vi "lxc.vi"() -> ()   [LabVIEW 2017]
uses:
  a005793b-7148-4334-a388-72e6511322f3.vi
panel:
  out "波形图表 4":cluster{dbl, "millisecond timer value":u32}[](graph)
  out "低温  5":bool
  out "高温 5":bool
  in  "停止 10":bool
  out "波形图 2":dbl[](graph)
  out "数组 2":string[](array[string])
  out "波形图表 3":dbl(graph)
  out "波形图表 2":cluster{"y":dbl, "y":dbl, dbl}(graph)
  in  "停止 9":bool
  out "高温 4":bool
  out "低温  4":bool
  out "低温  3":bool
  out "高温 3":bool
  in  "停止 8":bool
  out "波形图表":dbl(graph)
  out "实时温度":cluster{"y":dbl, "y":dbl, dbl}(graph)
  out "下限":bool
  out "上限":bool
  in  "停止 7":bool
  out "x-y":dbl
  in  "停止 6":bool
  in  "停止 5":bool
  out "高温 2":bool
  out "低温  2":bool
  in  "停止 4":bool
  out "已删除元素的数组子集":dbl[](array[numeric])
  out "已删除的部分":dbl[](array[numeric])
  out "重新排序":i32[](array[numeric]) caption="重排后数组"
  out "数组":i32[](array[numeric])
  in  "停止 3":bool
  out "温度 2":dbl
  out "数组 3":dbl[](array[numeric])
  out "温度":dbl
  in  "停止 2":bool
  out "低温":bool
  in  "停止":bool
  out "高温":bool
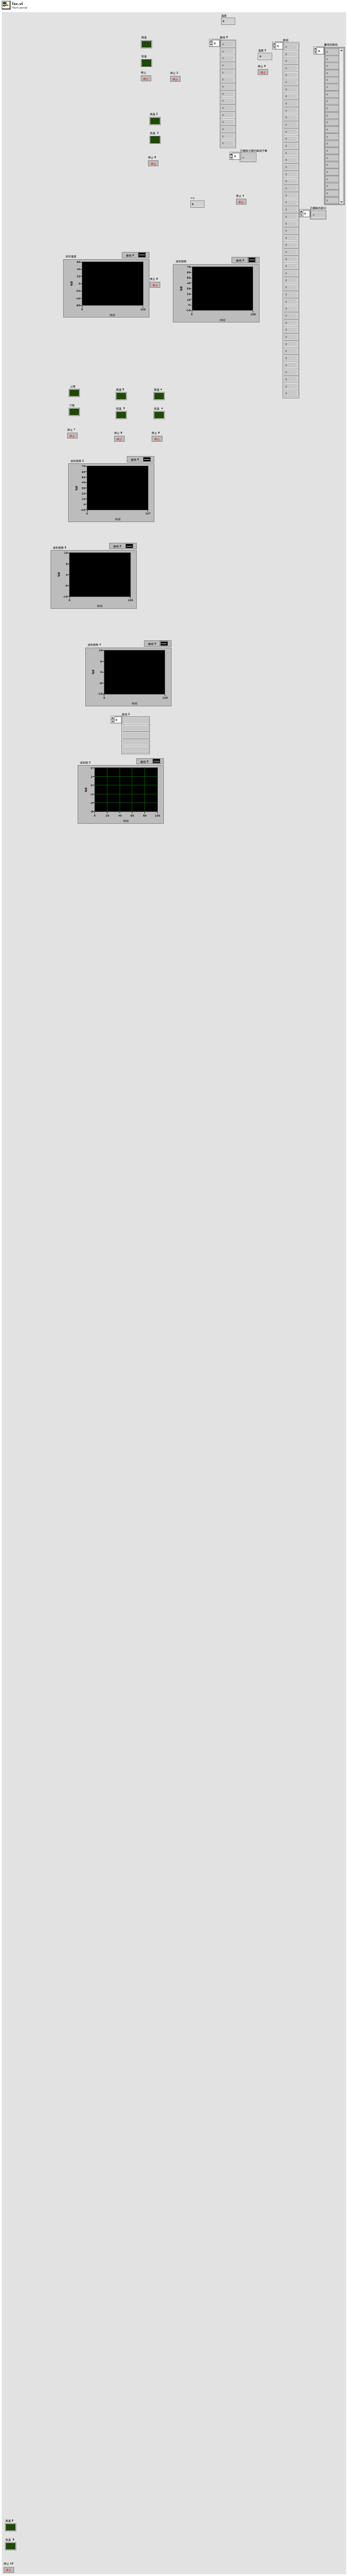
[diagram p1: front panel]
types:
  T1 = enum16{"open", "replace", "create", "open or create", "replace or create", "replace or create with confirmation"}
  T2 = typedef "控件 1.ctl" = i32
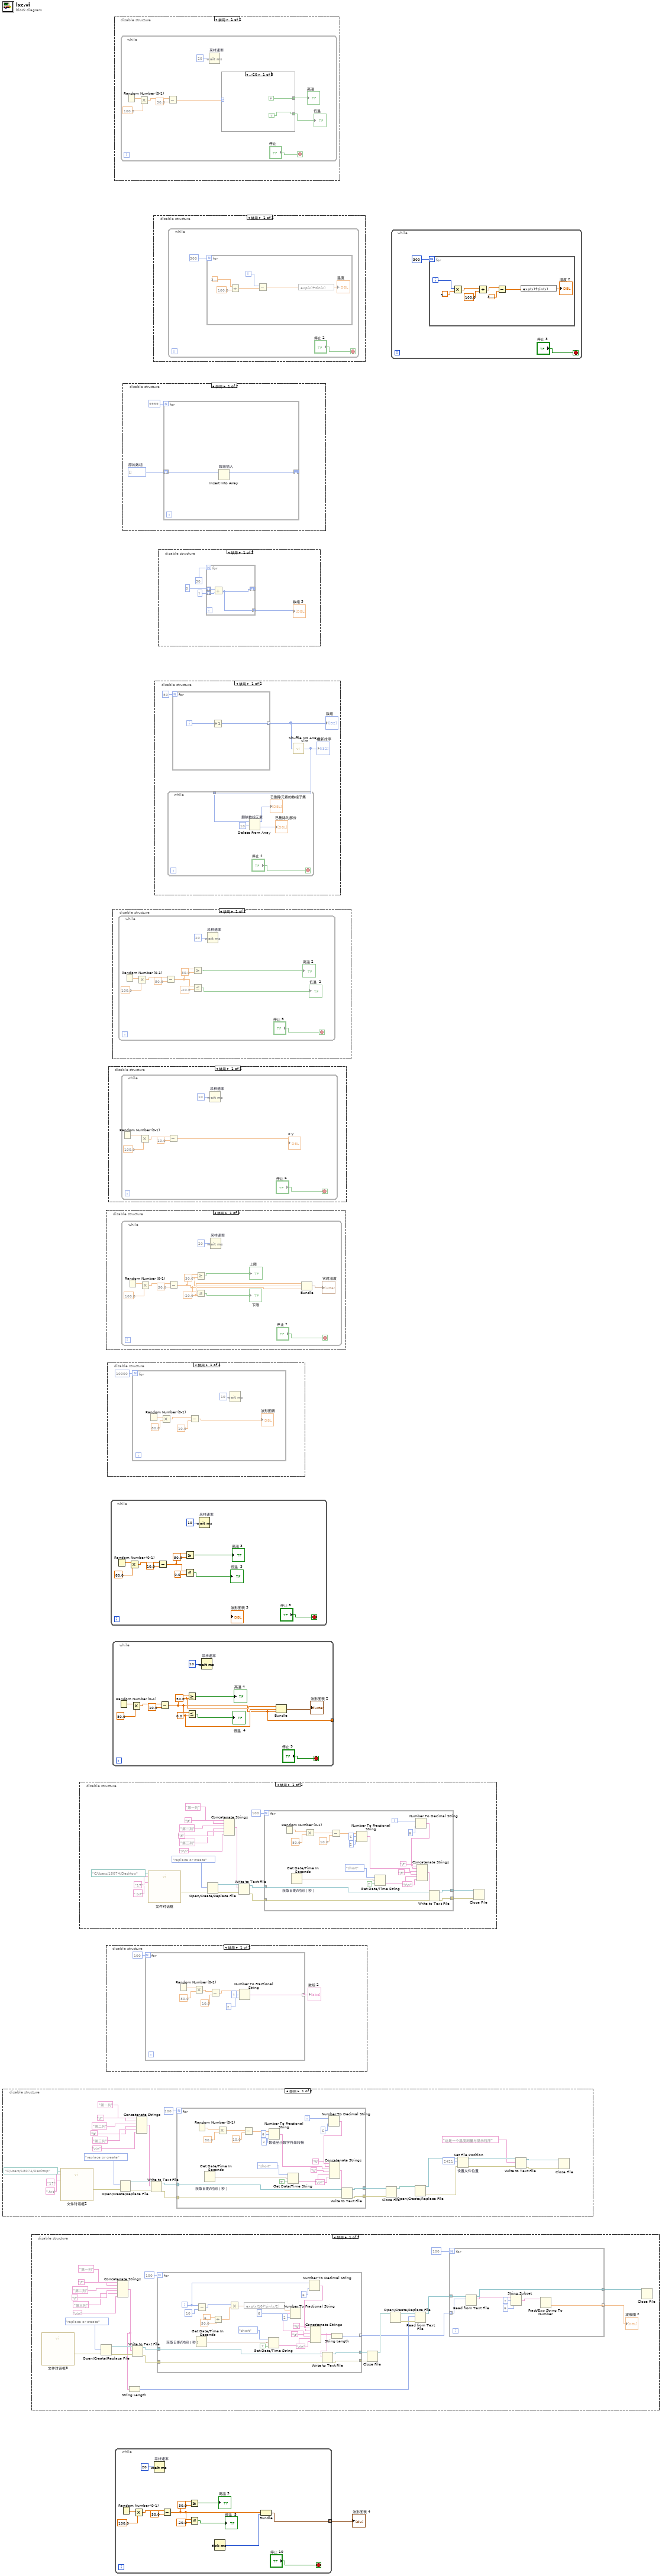
[diagram p0: block diagram]
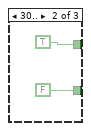
[diagram p14: hidden frame]
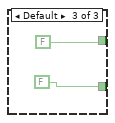
[diagram p15: hidden frame]
diagram:
  n1 = disable-structure shown="禁用" {
    frame Disabled {
      n2 = call "文件对话框2"("start path"=path "C:/Users/18074/Desktop", "default name"="17", "pattern (all files)"=".txt") -> ("error out"=w16:errorcluster)  [unwired: 9 in, 3 out]
      n3 = Open/Create/Replace File(error in=w16, operation (0:open)=T1."replace or create" ("操作(0:open)")) -> (refnum out=w17:refnum<file>, error out=w18:errorcluster)  [unwired: 4 in, 1 out]
      n4 = Concatenate Strings("第一列" ("字符串"), "\t", "第二列" ("字符串"), "\t", "第三列" ("字符串"), "\r\n") -> (w23:string)
      n5 = Write to Text File(file (use dialog)=w17, text=w23, error in=w18) -> (refnum out=w20:refnum<file>, error out=w19:errorcluster)  [unwired: 1 in, 1 out]
      n6 = for {
        N: 100 -> [_]
        tunnel: w20 -> [w48]
        tunnel: w19 -> [w47]
        tunnel: [w37] -> w21
        tunnel: [w36] -> w22
        i -> [w42]
        n7 = Random Number (0-1)() -> (number: 0 to 1=w52:dbl)
        n8 = Get Date/Time In Seconds "获取日期/时间（秒）"() -> (seconds since 1Jan1904=w32:timestamp)
        n9 = Multiply(x=w52, y=80.0) -> (x*y=w50:dbl)
        n10 = Subtract(x=w50, y=10.0) -> (x-y=w45:dbl)
        n11 = Number To Fractional String "数值至小数字符串转换"(number=w45, width (-)=i16 6 ("宽度(-)"), precision (6)=i16 2 ("精度(6)")) -> (F-format string=w39:string)  [unwired: 1 in]
        n12 = Get Date/Time String(date format (0)=enum16{"short", "long", "abbreviated"}."short" ("日期格式(0)"), seconds (now)=w32, want seconds? (F)=TRUE ("UTC格式")) -> (time string=w31:string)  [unwired: 1 out]
        n13 = Number To Decimal String(number=w42, width (-)=i16 6 ("宽度(-)")) -> (decimal integer string=w41:string)
        n14 = Concatenate Strings(w41, "\t", w39, "\t", w31, "\r\n") -> (w35:string)
        n15 = Write to Text File(file (use dialog)=w48, text=w35, error in=w47) -> (refnum out=w37:refnum<file>, error out=w36:errorcluster)  [unwired: 1 in, 1 out]
      }
      n16 = Close File(refnum=w21, error in=w22) -> (path=w10:path)  [unwired: 1 out]
      n17 = Open/Create/Replace File(file path (use dialog)=w10) -> (refnum out=w9:refnum<file>, error out=w8:errorcluster)  [unwired: 5 in, 1 out]
      n18 = Set File Position "设置文件位置"(offset (in bytes) (0)=i64 2421 ("偏移量（字节）（0）"), refnum=w9, error in=w8) -> (refnum out=w7:refnum<file>, error out=w6:errorcluster)  [unwired: 1 in]
      n19 = Write to Text File(file (use dialog)=w7, text="这是一个温度测量与显示程序" ("文本"), error in=w6) -> (refnum out=w4:refnum<file>, error out=w3:errorcluster)  [unwired: 1 in, 1 out]
      n20 = Close File(refnum=w4, error in=w3) -> ()  [unwired: 2 out]
    }
    frame Enabled {
    }
  }
  n21 = disable-structure shown="禁用" {
    frame Disabled {
      n22 = call "文件对话框3"() -> ("error out"=w75:errorcluster)  [unwired: 12 in, 3 out]
      n23 = Open/Create/Replace File(error in=w75, operation (0:open)=T1."replace or create" ("操作(0:open)")) -> (refnum out=w74:refnum<file>, error out=w73:errorcluster)  [unwired: 4 in, 1 out]
      n24 = Concatenate Strings("第一列" ("字符串"), "\t", "第二列" ("字符串"), "\t", "第三列" ("字符串"), "\r\n") -> (w62:string)
      n25 = String Length(string=w62) -> (length=w57:i32)
      n26 = Write to Text File(file (use dialog)=w74, text=w62, error in=w73) -> (refnum out=w71:refnum<file>, error out=w72:errorcluster)  [unwired: 1 in, 1 out]
      n27 = for {
        N: 100 -> [_]
        tunnel: w71 -> [w111]
        tunnel: w72 -> [w110]
        tunnel: [w104] -> w70
        tunnel: [w103] -> w69
        tunnel: [w88] -> w55 mode=indexing
        i -> [w86]
        n28 = Get Date/Time In Seconds "获取日期/时间（秒）"() -> (seconds since 1Jan1904=w100:timestamp)
        n29 = Subtract(x=w86, y=10) -> (x-y=w96:i32)
        n30 = Divide(x=6.283185307179586, y=50.0) -> (x/y=w93:dbl)
        n31 = Multiply(x=w96, y=w93) -> (x*y=w92:dbl)
        n32 = expression code="exp(x/10)*sin(x/2)"(w92) -> (w91:dbl)
        n33 = Get Date/Time String(date format (0)=enum16{"short", "long", "abbreviated"}."short" ("日期格式(0)"), seconds (now)=w100, want seconds? (F)=TRUE ("UTC格式")) -> (time string=w99:string)  [unwired: 1 out]
        n34 = Number To Fractional String ("数值至小数字符串转换")(number=w91, width (-)=i16 6 ("宽度(-)"), precision (6)=i16 2 ("精度(6)")) -> (F-format string=w106:string)  [unwired: 1 in]
        n35 = Number To Decimal String(number=w86, width (-)=i16 6 ("宽度(-)")) -> (decimal integer string=w108:string)
        n36 = Concatenate Strings(w108, "\t", w106, "\t", w99, "\r\n") -> (w87:string)
        n37 = Write to Text File(file (use dialog)=w111, text=w87, error in=w110) -> (refnum out=w104:refnum<file>, error out=w103:errorcluster)  [unwired: 1 in, 1 out]
        n38 = String Length(string=w87) -> (length=w88:i32)
      }
      n39 = Close File(refnum=w70, error in=w69) -> (path=w60:path)  [unwired: 1 out]
      n40 = Open/Create/Replace File(file path (use dialog)=w60) -> (refnum out=w58:refnum<file>, error out=w59:errorcluster)  [unwired: 5 in, 1 out]
      n41 = Read from Text File(file (use dialog)=w58, count=w57, error in=w59) -> (refnum out=w56:refnum<file>)  [unwired: 1 in, 3 out]
      n42 = for {
        N: 100 -> [_]
        tunnel: w56 -> [w85]
        tunnel: w55 -> [w84] mode=indexing
        tunnel: [w80] -> w54
        tunnel: [w78] -> w53 mode=indexing
        n43 = Read from Text File(file (use dialog)=w85, count=w84) -> (refnum out=w80:refnum<file>, text=w83:string)  [unwired: 2 in, 2 out]
        n44 = String Subset(string=w83, offset (0)=7 ("偏移量(0)"), length (rest)=6 ("长度（剩余）")) -> (substring=w79:string)
        n45 = Fract/Exp String To Number(string=w79) -> (number=w78:dbl)  [unwired: 3 in, 1 out]
      }
      "波形图 2" <- w53
      n46 = Close File(refnum=w54) -> ()  [unwired: 1 in, 2 out]
    }
    frame Enabled {
    }
  }
  n47 = disable-structure shown="禁用" {
    frame Disabled {
      n48 = call "文件对话框"("start path"=path "C:/Users/18074/Desktop", "default name"="17", "pattern (all files)"=".txt") -> ("error out"=w125:errorcluster)  [unwired: 9 in, 3 out]
      n49 = Open/Create/Replace File(error in=w125, operation (0:open)=T1."replace or create" ("操作(0:open)")) -> (refnum out=w124:refnum<file>, error out=w123:errorcluster)  [unwired: 4 in, 1 out]
      n50 = Concatenate Strings("第一列" ("字符串"), "\t", "第二列" ("字符串"), "\t", "第三列" ("字符串"), "\r\n") -> (w118:string)
      n51 = Write to Text File(file (use dialog)=w124, text=w118, error in=w123) -> (refnum out=w121:refnum<file>, error out=w122:errorcluster)  [unwired: 1 in, 1 out]
      n52 = for {
        N: 100 -> [_]
        tunnel: w121 -> [w149]
        tunnel: w122 -> [w148]
        tunnel: [w138] -> w120
        tunnel: [w137] -> w119
        i -> [w143]
        n53 = Random Number (0-1)() -> (number: 0 to 1=w153:dbl)
        n54 = Get Date/Time In Seconds "获取日期/时间（秒）"() -> (seconds since 1Jan1904=w133:timestamp)
        n55 = Multiply(x=w153, y=80.0) -> (x*y=w151:dbl)
        n56 = Subtract(x=w151, y=10.0) -> (x-y=w146:dbl)
        n57 = Number To Fractional String(number=w146, width (-)=i16 6 ("宽度(-)"), precision (6)=i16 2 ("精度(6)")) -> (F-format string=w140:string)  [unwired: 1 in]
        n58 = Get Date/Time String(date format (0)=enum16{"short", "long", "abbreviated"}."short" ("日期格式(0)"), seconds (now)=w133, want seconds? (F)=TRUE ("UTC格式")) -> (time string=w132:string)  [unwired: 1 out]
        n59 = Number To Decimal String(number=w143, width (-)=i16 6 ("宽度(-)")) -> (decimal integer string=w142:string)
        n60 = Concatenate Strings(w142, "\t", w140, "\t", w132, "\r\n") -> (w136:string)
        n61 = Write to Text File(file (use dialog)=w149, text=w136, error in=w148) -> (refnum out=w138:refnum<file>, error out=w137:errorcluster)  [unwired: 1 in, 1 out]
      }
      n62 = Close File(refnum=w120, error in=w119) -> ()  [unwired: 2 out]
    }
    frame Enabled {
    }
  }
  n63 = disable-structure shown="禁用" {
    frame Disabled {
      n64 = for {
        N: 100 -> [_]
        tunnel: [w156] -> w154 mode=indexing
        n65 = Random Number (0-1)() -> (number: 0 to 1=w163:dbl)
        n66 = Multiply(x=w163, y=80.0) -> (x*y=w161:dbl)
        n67 = Subtract(x=w161, y=10.0) -> (x-y=w159:dbl)
        n68 = Number To Fractional String(number=w159, width (-)=i16 4 ("宽度(-)"), precision (6)=i16 2 ("精度(6)")) -> (F-format string=w156:string)  [unwired: 1 in]
      }
      "数组 2" <- w154
    }
    frame Enabled {
    }
  }
  n69 = disable-structure shown="禁用" {
    frame Disabled {
      n70 = while {
        stop <- "停止 7" stop-if-true
        w167 = -20.0 ("y")
        w166 = 30.0 ("y")
        n71 = Random Number (0-1)() -> (number: 0 to 1=w175:dbl)
        n72 = Multiply(x=w175, y=100.0) -> (x*y=w173:dbl)
        n73 = Subtract(x=w173, y=50.0) -> (x-y=w165:dbl)
        n74 = Greater Or Equal?(x=w165, y=w166) -> (x >= y?=→"上限":bool)
        n75 = Less Or Equal?(x=w165, y=w167) -> (x <= y?=→"下限":bool)
        n76 = Wait (ms) "采样速率"(milliseconds to wait=u32 20 ("等待时间（毫秒）")) -> ()  [unwired: 1 out]
        n77 = Bundle("y"=w167, "y"=w166, w165) -> (→"实时温度":cluster{"y":dbl, "y":dbl, dbl})  [unwired: 1 in]
      }
    }
    frame Enabled {
    }
  }
  n78 = disable-structure shown="禁用" {
    frame Disabled {
      n79 = for {
        N: 10000 -> [_]
        n80 = Random Number (0-1)() -> (number: 0 to 1=w180:dbl)
        n81 = Multiply(x=w180, y=80.0) -> (x*y=w181:dbl)
        n82 = Subtract(x=w181, y=10.0) -> (x-y=→"波形图表":dbl)
        n83 = Wait (ms)(milliseconds to wait=u32 10 ("等待时间（毫秒）")) -> ()  [unwired: 1 out]
      }
    }
    frame Enabled {
    }
  }
  n84 = disable-structure shown="禁用" {
    frame Disabled {
      n85 = while {
        stop <- "停止 6" stop-if-true
        n86 = Random Number (0-1)() -> (number: 0 to 1=w189:dbl)
        n87 = Multiply(x=w189, y=100.0) -> (x*y=w187:dbl)
        n88 = Subtract(x=w187, y=10.0) -> (x-y=→"x-y":dbl)
        n89 = Wait (ms) "采样速率"(milliseconds to wait=u32 10 ("等待时间（毫秒）")) -> ()  [unwired: 1 out]
      }
    }
    frame Enabled {
    }
  }
  n90 = while {
    stop <- "停止 8" stop-if-true
    n91 = Random Number (0-1)() -> (number: 0 to 1=w200:dbl)
    n92 = Multiply(x=w200, y=80.0) -> (x*y=w198:dbl)
    n93 = Subtract(x=w198, y=10.0) -> (x-y=w194:dbl)
    n94 = Greater Or Equal?(x=w194, y=50.0) -> (x >= y?=→"高温 3":bool)
    n95 = Less Or Equal?(x=w194, y=0.0) -> (x <= y?=→"低温  3":bool)
    n96 = Wait (ms) "采样速率"(milliseconds to wait=u32 10 ("等待时间（毫秒）")) -> ()  [unwired: 1 out]
  }
  n97 = disable-structure shown="禁用" {
    frame Disabled {
      n98 = while {
        stop <- "停止 5" stop-if-true
        n99 = Random Number (0-1)() -> (number: 0 to 1=w211:dbl)
        n100 = Multiply(x=w211, y=100.0) -> (x*y=w209:dbl)
        n101 = Subtract(x=w209, y=50.0) -> (x-y=w205:dbl)
        n102 = Greater Or Equal?(x=w205, y=30.0) -> (x >= y?=→"高温 2":bool)
        n103 = Less Or Equal?(x=w205, y=-20.0) -> (x <= y?=→"低温  2":bool)
        n104 = Wait (ms) "采样速率"(milliseconds to wait=u32 20 ("等待时间（毫秒）")) -> ()  [unwired: 1 out]
      }
    }
    frame Enabled {
    }
  }
  n105 = while {
    tunnel: [w212] -> _
    stop <- "停止 9" stop-if-true
    w214 = 0.0 ("y")
    w215 = 50.0 ("y")
    n106 = Random Number (0-1)() -> (number: 0 to 1=w223:dbl)
    n107 = Multiply(x=w223, y=80.0) -> (x*y=w221:dbl)
    n108 = Subtract(x=w221, y=10.0) -> (x-y=w212:dbl)
    n109 = Greater Or Equal?(x=w212, y=w215) -> (x >= y?=→"高温 4":bool)
    n110 = Less Or Equal?(x=w212, y=w214) -> (x <= y?=→"低温  4":bool)
    n111 = Wait (ms) "采样速率"(milliseconds to wait=u32 10 ("等待时间（毫秒）")) -> ()  [unwired: 1 out]
    n112 = Bundle("y"=w215, "y"=w214, w212) -> (→"波形图表 2":cluster{"y":dbl, "y":dbl, dbl})  [unwired: 1 in]
  }
  n113 = disable-structure shown="禁用" {
    frame Disabled {
      n114 = while {
        stop <- "停止" stop-if-true
        n115 = Random Number (0-1)() -> (number: 0 to 1=w232:dbl)
        n116 = Multiply(x=w232, y=100.0) -> (x*y=w230:dbl)
        n117 = Subtract(x=w230, y=50.0) -> (x-y=w227:dbl)
        n118 = Wait (ms) "采样速率"(milliseconds to wait=u32 20 ("等待时间（毫秒）")) -> ()  [unwired: 1 out]
        n119 = case shown="..-20" w227 {
          tunnel: [FALSE TRUE FALSE] -> w225
          tunnel: [TRUE FALSE FALSE] -> w224
          frame ..-20 {
          }
          frame 30.. {
          }
          frame Default {
          }
        }
        "高温" <- w225
        "低温" <- w224
      }
    }
    frame Enabled {
    }
  }
  n120 = while {
    tunnel: [w239] -> w1 mode=indexing
    stop <- "停止 10" stop-if-true
    n121 = Random Number (0-1)() -> (number: 0 to 1=w251:dbl)
    n122 = Multiply(x=w251, y=100.0) -> (x*y=w249:dbl)
    n123 = Wait (ms) "采样速率"(milliseconds to wait=u32 20 ("等待时间（毫秒）")) -> ()  [unwired: 1 out]
    n124 = Subtract(x=w249, y=50.0) -> (x-y=w241:dbl)
    n125 = Greater Or Equal?(x=w241, y=30.0) -> (x >= y?=→"高温 5":bool)
    n126 = Less Or Equal?(x=w241, y=-20.0) -> (x <= y?=→"低温  5":bool)
    n127 = Tick Count (ms)() -> (millisecond timer value=w240:u32)
    n128 = Bundle(w241, "millisecond timer value"=w240) -> (w239:cluster{dbl, "millisecond timer value":u32})  [unwired: 1 in]
  }
  "波形图表 4" <- w1
  n129 = disable-structure shown="禁用" {
    frame Disabled {
      w252 = i32[] []  # 原始数组
      n130 = for {
        N: 9999 -> [_]
        shift-right: [w254] -> _
        shift-left: w252 -> [w255]
        n131 = Insert Into Array "数组插入"(array=w255) -> (w254:i32[])  [unwired: 2 in]
      }
    }
    frame Enabled {
    }
  }
  n132 = disable-structure shown="禁用" {
    frame Disabled {
      n133 = while {
        stop <- "停止 2" stop-if-true
        n134 = for {
          N: 300 -> [_]
          i -> [w261]
          n135 = Divide(x=3.141592653589793, y=100.0) -> (x/y=w260:dbl)
          n136 = Subtract(x=w261, y=w260) -> (x-y=w259:dbl)
          n137 = expression code="exp(x)+sin(x)"(w259) -> (→"温度":dbl)
        }
      }
    }
    frame Enabled {
    }
  }
  n138 = disable-structure shown="禁用" {
    frame Disabled {
      n139 = for {
        N: 50 -> [_]
        tunnel: [w272] -> w265 mode=indexing
        i -> [w273]
        n140 = Increment(x=w273) -> (x+1=w272:i32)
      }
      "数组" <- w265
      n141 = call "Shuffle 1D Array.vim"("array"=w265) -> ("shuffled array"=w264:i32[])  [unwired: 4 in]
      "重新排序" <- w264
      n142 = while {
        tunnel: w264 -> [w271]
        stop <- "停止 4" stop-if-true
        n143 = Delete From Array "删除数组元素"(array=w271, length=10 ("长度")) -> (deleted portion=→"已删除的部分":i32[], array with subset deleted=→"已删除元素的数组子集":i32[])  [unwired: 1 in]
      }
    }
    frame Enabled {
    }
  }
  n144 = disable-structure shown="禁用" {
    frame Disabled {
      n145 = for {
        N: T2 50 -> [_]
        shift-right: [w278] -> _
        shift-left: T2 0 -> [w280]
        shift-left: T2 1 -> [w279]
        tunnel: [w278] -> w276 mode=indexing
        n146 = Add(x=w280, y=w279) -> (x+y=w278:T2)
      }
      "数组 3" <- w276
    }
    frame Enabled {
    }
  }
  n147 = while {
    stop <- "停止 3" stop-if-true
    n148 = for {
      N: 300 -> [_]
      i -> [w289]
      n149 = Multiply(x=w289, y=3.141592653589793) -> (x*y=w287:dbl)
      n150 = Divide(x=w287, y=100.0) -> (x/y=w285:dbl)
      n151 = Subtract(x=w285, y=3.141592653589793) -> (x-y=w283:dbl)
      n152 = expression code="exp(x)+sin(x)"(w283) -> (→"温度 2":dbl)
    }
  }
